vi "Convert Status Code to Status Symbol.vi"(8 "error in (no error)":errorcluster, 11 "Status Code":i32) -> (0 "error out":errorcluster, 3 "Status String":string)   [LabVIEW 2018, in "PicoScope 3000a.lvlib" / "PicoScope 3000a.lvclass"]
uses:
  PicoScope 3000a.lvclass
  Custom Controls/Status Array.ctl
  Custom Controls/Status Symbol.ctl
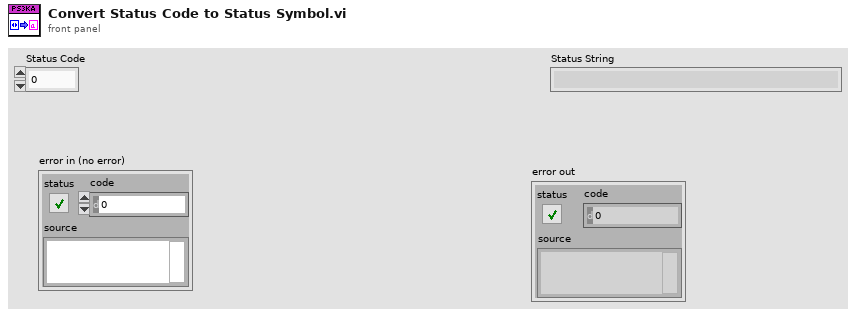
[diagram p1: front panel]
types:
  T1 = typedef "PicoScope 3000a.lvlib/PicoScope 3000a.lvclass/Status Array.ctl" = cluster{"Code (HEX)":i32, "Status":T2}[]
  T2 = typedef "PicoScope 3000a.lvlib/PicoScope 3000a.lvclass/Status Symbol.ctl" = enum16{"PICO_OK ", "PICO_MAX_UNITS_OPENED", "PICO_MEMORY_FAIL", "PICO_NOT_FOUND ", "PICO_FW_FAIL ", "PICO_OPEN_OPERATION_IN_PROGRESS", "PICO_OPERATION_FAILED", "PICO_NOT_RESPONDING", "PICO_CONFIG_FAIL ", "PICO_KERNEL_DRIVER_TOO_OLD ", "PICO_EEPROM_CORRUPT", "PICO_OS_NOT_SUPPORTED ", "PICO_INVALID_HANDLE ", "PICO_INVALID_PARAMETER", "PICO_INVALID_TIMEBASE ", "PICO_INVALID_VOLTAGE_RANGE ", "PICO_INVALID_CHANNEL ", "PICO_INVALID_TRIGGER_CHANNEL", "PICO_INVALID_CONDITION_CHANNEL ", "PICO_NO_SIGNAL_GENERATOR ", "PICO_STREAMING_FAILED ", "PICO_BLOCK_MODE_FAILED ", "PICO_NULL_PARAMETER ", "PICO_DATA_NOT_AVAILABLE ", "PICO_STRING_BUFFER_TOO_SMALL ", "PICO_ETS_NOT_SUPPORTED ", "PICO_AUTO_TRIGGER_TIME_TOO_SHORT ", "PICO_BUFFER_STALL ", "PICO_TOO_MANY_SAMPLES ", "PICO_TOO_MANY_SEGMENTS ", "PICO_PULSE_WIDTH_QUALIFIER ", "PICO_DELAY ", "PICO_SOURCE_DETAILS ", "PICO_CONDITIONS ", "PICO_USER_CALLBACK ", "PICO_DEVICE_SAMPLING ", "PICO_NO_SAMPLES_AVAILABLE ", "PICO_SEGMENT_OUT_OF_RANGE ", "PICO_BUSY ", "PICO_STARTINDEX_INVALID ", "PICO_INVALID_INFO ", "PICO_INFO_UNAVAILABLE ", "PICO_INVALID_SAMPLE_INTERVAL ", "PICO_TRIGGER_ERROR ", "PICO_MEMORY ", "PICO_SIG_GEN_PARAM ", "PICO_SHOTS_SWEEPS_WARNING ", "PICO_WARNING_EXT_THRESHOLD_CONFLICT ", "PICO_SIGGEN_OUTPUT_OVER_VOLTAGE ", "PICO_DELAY_NULL", "PICO_INVALID_BUFFER ", "PICO_SIGGEN_OFFSET_VOLTAGE ", "PICO_SIGGEN_PK_TO_PK ", "PICO_CANCELLED ", "PICO_SEGMENT_NOT_USED ", "PICO_INVALID_CALL ", "PICO_NOT_USED ", "PICO_INVALID_SAMPLERATIO ", "PICO_INVALID_STATE ", "PICO_NOT_ENOUGH_SEGMENTS ", "PICO_DRIVER_FUNCTION ", "PICO_RESERVED ", "PICO_INVALID_COUPLING ", "PICO_BUFFERS_NOT_SET ", "PICO_RATIO_MODE_NOT_SUPPORTED ", "PICO_INVALID_TRIGGER_PROPERTY", "PICO_INTERFACE_NOT_CONNECTED ", "PICO_SIGGEN_WAVEFORM_SETUP_FAILED ", "PICO_FPGA_FAIL ", "PICO_POWER_MANAGER ", "PICO_INVALID_ANALOGUE_OFFSET ", "PICO_PLL_LOCK_FAILED ", "PICO_ANALOG_BOARD ", "PICO_CONFIG_FAIL_AWG ", "PICO_INITIALISE_FPGA ", "PICO_EXTERNAL_FREQUENCY_INVALID ", "PICO_CLOCK_CHANGE_ERROR ", "PICO_TRIGGER_AND_EXTERNAL_CLOCK_CLASH ", "PICO_PWQ_AND_EXTERNAL_CLOCK_CLASH ", "PICO_UNABLE_TO_OPEN_SCALING_FILE ", "PICO_MEMORY_CLOCK_FREQUENCY ", "PICO_I2C_NOT_RESPONDING ", "PICO_NO_CAPTURES_AVAILABLE ", "PICO_NOT_USED_IN_THIS_CAPTURE_MODE ", "PICO_GET_DATA_ACTIVE ", "PICO_IP_NETWORKED ", "PICO_INVALID_IP_ADDRESS ", "PICO_IPSOCKET_FAILED ", "PICO_IPSOCKET_TIMEDOUT ", "PICO_SETTINGS_FAILED ", "PICO_NETWORK_FAILED ", "PICO_WS2_32_DLL_NOT_LOADED ", "PICO_INVALID_IP_PORT ", "PICO_COUPLING_NOT_SUPPORTED ", "PICO_BANDWIDTH_NOT_SUPPORTED ", "PICO_INVALID_BANDWIDTH ", "PICO_AWG_NOT_SUPPORTED ", "PICO_ETS_NOT_RUNNING ", "PICO_SIG_GEN_WHITENOISE_NOT_SUPPORTED ", "PICO_SIG_GEN_WAVETYPE_NOT_SUPPORTED ", "PICO_INVALID_DIGITAL_PORT ", "PICO_INVALID_DIGITAL_CHANNEL ", "PICO_INVALID_DIGITAL_TRIGGER_DIRECTION ", "PICO_SIG_GEN_PRBS_NOT_SUPPORTED ", "PICO_ETS_NOT_AVAILABLE_WITH_LOGIC_CHANNELS ", "PICO_WARNING_REPEAT_VALUE ", "PICO_POWER_SUPPLY_CONNECTED ", "PICO_POWER_SUPPLY_NOT_CONNECTED ", "PICO_POWER_SUPPLY_REQUEST_INVALID ", "PICO_POWER_SUPPLY_UNDERVOLTAGE ", "PICO_CAPTURING_DATA ", "PICO_USB3_0_DEVICE_NON_USB3_0_PORT"}
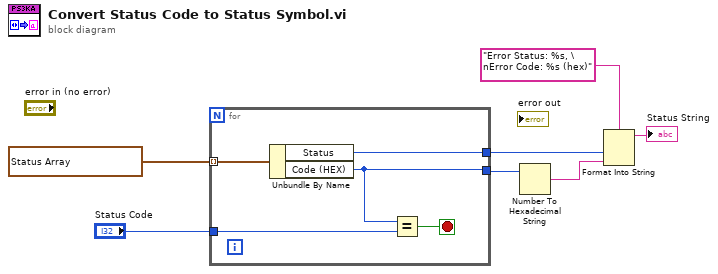
[diagram p0: block diagram]
diagram:
  n1 = for {
    tunnel: T1 [{"Code (HEX)"=0, "Status"=enum."PICO_OK "}, {"Code (HEX)"=1, "Status"=enum."PICO_MAX_UNITS_OPENED"}, {"Code (HEX)"=2, "Status"=enum."PICO_MEMORY_FAIL"}, {"Code (HEX)"=3, "Status"=enum."PICO_NOT_FOUND "}, {"Code (HEX)"=4, "Status"=enum."PICO_FW_FAIL "}, {"Code (HEX)"=5, "Status"=enum."PICO_OPEN_OPERATION_IN_PROGRESS"}, {"Code (HEX)"=6, "Status"=enum."PICO_OPERATION_FAILED"}, {"Code (HEX)"=7, "Status"=enum."PICO_NOT_RESPONDING"}, {"Code (HEX)"=8, "Status"=enum."PICO_CONFIG_FAIL "}, {"Code (HEX)"=9, "Status"=enum."PICO_KERNEL_DRIVER_TOO_OLD "}, {"Code (HEX)"=10, "Status"=enum."PICO_EEPROM_CORRUPT"}, {"Code (HEX)"=11, "Status"=enum."PICO_OS_NOT_SUPPORTED "}, {"Code (HEX)"=12, "Status"=enum."PICO_INVALID_HANDLE "}, {"Code (HEX)"=13, "Status"=enum."PICO_INVALID_PARAMETER"}, {"Code (HEX)"=14, "Status"=enum."PICO_INVALID_TIMEBASE "}, {"Code (HEX)"=15, "Status"=enum."PICO_INVALID_VOLTAGE_RANGE "}, {"Code (HEX)"=16, "Status"=enum."PICO_INVALID_CHANNEL "}, {"Code (HEX)"=17, "Status"=enum."PICO_INVALID_TRIGGER_CHANNEL"}, {"Code (HEX)"=18, "Status"=enum."PICO_INVALID_CONDITION_CHANNEL "}, {"Code (HEX)"=19, "Status"=enum."PICO_NO_SIGNAL_GENERATOR "}, {"Code (HEX)"=20, "Status"=enum."PICO_STREAMING_FAILED "}, {"Code (HEX)"=21, "Status"=enum."PICO_BLOCK_MODE_FAILED "}, {"Code (HEX)"=22, "Status"=enum."PICO_NULL_PARAMETER "}, {"Code (HEX)"=24, "Status"=enum."PICO_DATA_NOT_AVAILABLE "}, {"Code (HEX)"=25, "Status"=enum."PICO_STRING_BUFFER_TOO_SMALL "}, {"Code (HEX)"=26, "Status"=enum."PICO_ETS_NOT_SUPPORTED "}, {"Code (HEX)"=27, "Status"=enum."PICO_AUTO_TRIGGER_TIME_TOO_SHORT "}, {"Code (HEX)"=28, "Status"=enum."PICO_BUFFER_STALL "}, {"Code (HEX)"=29, "Status"=enum."PICO_TOO_MANY_SAMPLES "}, {"Code (HEX)"=30, "Status"=enum."PICO_TOO_MANY_SEGMENTS "}, {"Code (HEX)"=31, "Status"=enum."PICO_PULSE_WIDTH_QUALIFIER "}, {"Code (HEX)"=32, "Status"=enum."PICO_DELAY "}, {"Code (HEX)"=33, "Status"=enum."PICO_SOURCE_DETAILS "}, {"Code (HEX)"=34, "Status"=enum."PICO_CONDITIONS "}, {"Code (HEX)"=35, "Status"=enum."PICO_USER_CALLBACK "}, {"Code (HEX)"=36, "Status"=enum."PICO_DEVICE_SAMPLING "}, {"Code (HEX)"=37, "Status"=enum."PICO_NO_SAMPLES_AVAILABLE "}, {"Code (HEX)"=38, "Status"=enum."PICO_SEGMENT_OUT_OF_RANGE "}, {"Code (HEX)"=39, "Status"=enum."PICO_BUSY "}, {"Code (HEX)"=40, "Status"=enum."PICO_STARTINDEX_INVALID "}, {"Code (HEX)"=41, "Status"=enum."PICO_INVALID_INFO "}, {"Code (HEX)"=42, "Status"=enum."PICO_INFO_UNAVAILABLE "}, {"Code (HEX)"=43, "Status"=enum."PICO_INVALID_SAMPLE_INTERVAL "}, {"Code (HEX)"=44, "Status"=enum."PICO_TRIGGER_ERROR "}, {"Code (HEX)"=45, "Status"=enum."PICO_MEMORY "}, {"Code (HEX)"=46, "Status"=enum."PICO_SIG_GEN_PARAM "}, {"Code (HEX)"=47, "Status"=enum."PICO_SHOTS_SWEEPS_WARNING "}, {"Code (HEX)"=51, "Status"=enum."PICO_WARNING_EXT_THRESHOLD_CONFLICT "}, {"Code (HEX)"=53, "Status"=enum."PICO_SIGGEN_OUTPUT_OVER_VOLTAGE "}, {"Code (HEX)"=54, "Status"=enum."PICO_DELAY_NULL"}, {"Code (HEX)"=55, "Status"=enum."PICO_INVALID_BUFFER "}, {"Code (HEX)"=56, "Status"=enum."PICO_SIGGEN_OFFSET_VOLTAGE "}, {"Code (HEX)"=57, "Status"=enum."PICO_SIGGEN_PK_TO_PK "}, {"Code (HEX)"=58, "Status"=enum."PICO_CANCELLED "}, {"Code (HEX)"=59, "Status"=enum."PICO_SEGMENT_NOT_USED "}, {"Code (HEX)"=60, "Status"=enum."PICO_INVALID_CALL "}, {"Code (HEX)"=63, "Status"=enum."PICO_NOT_USED "}, {"Code (HEX)"=64, "Status"=enum."PICO_INVALID_SAMPLERATIO "}, {"Code (HEX)"=65, "Status"=enum."PICO_INVALID_STATE "}, {"Code (HEX)"=66, "Status"=enum."PICO_NOT_ENOUGH_SEGMENTS "}, {"Code (HEX)"=67, "Status"=enum."PICO_DRIVER_FUNCTION "}, {"Code (HEX)"=68, "Status"=enum."PICO_RESERVED "}, {"Code (HEX)"=69, "Status"=enum."PICO_INVALID_COUPLING "}, {"Code (HEX)"=70, "Status"=enum."PICO_BUFFERS_NOT_SET "}, {"Code (HEX)"=71, "Status"=enum."PICO_RATIO_MODE_NOT_SUPPORTED "}, {"Code (HEX)"=73, "Status"=enum."PICO_INVALID_TRIGGER_PROPERTY"}, {"Code (HEX)"=74, "Status"=enum."PICO_INTERFACE_NOT_CONNECTED "}, {"Code (HEX)"=77, "Status"=enum."PICO_SIGGEN_WAVEFORM_SETUP_FAILED "}, {"Code (HEX)"=78, "Status"=enum."PICO_FPGA_FAIL "}, {"Code (HEX)"=79, "Status"=enum."PICO_POWER_MANAGER "}, {"Code (HEX)"=80, "Status"=enum."PICO_INVALID_ANALOGUE_OFFSET "}, {"Code (HEX)"=81, "Status"=enum."PICO_PLL_LOCK_FAILED "}, {"Code (HEX)"=82, "Status"=enum."PICO_ANALOG_BOARD "}, {"Code (HEX)"=83, "Status"=enum."PICO_CONFIG_FAIL_AWG "}, {"Code (HEX)"=84, "Status"=enum."PICO_INITIALISE_FPGA "}, {"Code (HEX)"=86, "Status"=enum."PICO_EXTERNAL_FREQUENCY_INVALID "}, {"Code (HEX)"=87, "Status"=enum."PICO_CLOCK_CHANGE_ERROR "}, {"Code (HEX)"=88, "Status"=enum."PICO_TRIGGER_AND_EXTERNAL_CLOCK_CLASH "}, {"Code (HEX)"=89, "Status"=enum."PICO_PWQ_AND_EXTERNAL_CLOCK_CLASH "}, {"Code (HEX)"=90, "Status"=enum."PICO_UNABLE_TO_OPEN_SCALING_FILE "}, {"Code (HEX)"=91, "Status"=enum."PICO_MEMORY_CLOCK_FREQUENCY "}, {"Code (HEX)"=92, "Status"=enum."PICO_I2C_NOT_RESPONDING "}, {"Code (HEX)"=93, "Status"=enum."PICO_NO_CAPTURES_AVAILABLE "}, {"Code (HEX)"=94, "Status"=enum."PICO_NOT_USED_IN_THIS_CAPTURE_MODE "}, {"Code (HEX)"=259, "Status"=enum."PICO_GET_DATA_ACTIVE "}, {"Code (HEX)"=260, "Status"=enum."PICO_IP_NETWORKED "}, {"Code (HEX)"=261, "Status"=enum."PICO_INVALID_IP_ADDRESS "}, {"Code (HEX)"=262, "Status"=enum."PICO_IPSOCKET_FAILED "}, {"Code (HEX)"=263, "Status"=enum."PICO_IPSOCKET_TIMEDOUT "}, {"Code (HEX)"=264, "Status"=enum."PICO_SETTINGS_FAILED "}, {"Code (HEX)"=265, "Status"=enum."PICO_NETWORK_FAILED "}, {"Code (HEX)"=266, "Status"=enum."PICO_WS2_32_DLL_NOT_LOADED "}, {"Code (HEX)"=267, "Status"=enum."PICO_INVALID_IP_PORT "}, {"Code (HEX)"=268, "Status"=enum."PICO_COUPLING_NOT_SUPPORTED "}, {"Code (HEX)"=269, "Status"=enum."PICO_BANDWIDTH_NOT_SUPPORTED "}, {"Code (HEX)"=270, "Status"=enum."PICO_INVALID_BANDWIDTH "}, {"Code (HEX)"=271, "Status"=enum."PICO_AWG_NOT_SUPPORTED "}, {"Code (HEX)"=272, "Status"=enum."PICO_ETS_NOT_RUNNING "}, {"Code (HEX)"=273, "Status"=enum."PICO_SIG_GEN_WHITENOISE_NOT_SUPPORTED "}, {"Code (HEX)"=274, "Status"=enum."PICO_SIG_GEN_WAVETYPE_NOT_SUPPORTED "}, {"Code (HEX)"=275, "Status"=enum."PICO_INVALID_DIGITAL_PORT "}, {"Code (HEX)"=276, "Status"=enum."PICO_INVALID_DIGITAL_CHANNEL "}, {"Code (HEX)"=277, "Status"=enum."PICO_INVALID_DIGITAL_TRIGGER_DIRECTION "}, {"Code (HEX)"=278, "Status"=enum."PICO_SIG_GEN_PRBS_NOT_SUPPORTED "}, {"Code (HEX)"=279, "Status"=enum."PICO_ETS_NOT_AVAILABLE_WITH_LOGIC_CHANNELS "}, {"Code (HEX)"=280, "Status"=enum."PICO_WARNING_REPEAT_VALUE "}, {"Code (HEX)"=281, "Status"=enum."PICO_POWER_SUPPLY_CONNECTED "}, {"Code (HEX)"=282, "Status"=enum."PICO_POWER_SUPPLY_NOT_CONNECTED "}, {"Code (HEX)"=283, "Status"=enum."PICO_POWER_SUPPLY_REQUEST_INVALID "}, {"Code (HEX)"=284, "Status"=enum."PICO_POWER_SUPPLY_UNDERVOLTAGE "}, {"Code (HEX)"=285, "Status"=enum."PICO_CAPTURING_DATA "}, {"Code (HEX)"=286, "Status"=enum."PICO_USB3_0_DEVICE_NON_USB3_0_PORT"}] ("Status Array") -> [w12] mode=indexing
    tunnel: "Status Code" -> [w11]
    tunnel: [w9] -> w2
    tunnel: [w8] -> w4
    stop <- w10 stop-if-true
    n2 = Unbundle By Name(w12) -> ("Status"=w9:T2, "Code (HEX)"=w8:i32)
    n3 = Equal?(x=w8, y=w11) -> (x = y?=w10:bool)
  }
  n4 = Number To Hexadecimal String(2:w4) -> (0:w1:string)  [unwired: 1 in]
  n5 = Format Into String(format string="Error Status: %s, \nError Code: %s (hex)", w2, w1) -> (resulting string=→"Status String":string)  [unwired: 2 in, 1 out]
